vi "process mappings.vi"(4 "output dictionary":refnum<class "data dictionary.lvclass">, 6 "input dictionary":refnum<class "data dictionary.lvclass">, 8 "error in":errorcluster, 11 "modbus channels":refnum<class "Modbus Module Channel.lvclass">[](array[class])) -> (0 "error out":errorcluster, 2 "output accesses":T1[](array[typedef]), 3 "input accesses":T5[](array[typedef]))   [LabVIEW 2013, in "Modbus Slave runtime.lvclass"]
uses:
  Modbus Slave runtime.lvclass
  <vilib>/NI/Tag Bus/dictionary/data dictionary.lvclass
  bulk data access.ctl
  module channel/data bank type.ctl
  data mapping elements.ctl
  <vilib>/NI/Tag Bus/tag/Data Type.ctl
  output bulk data access.ctl
  module channel/Modbus Module Channel.lvclass
  <vilib>/NI/Tag Bus/tag/tag descriptor.lvclass
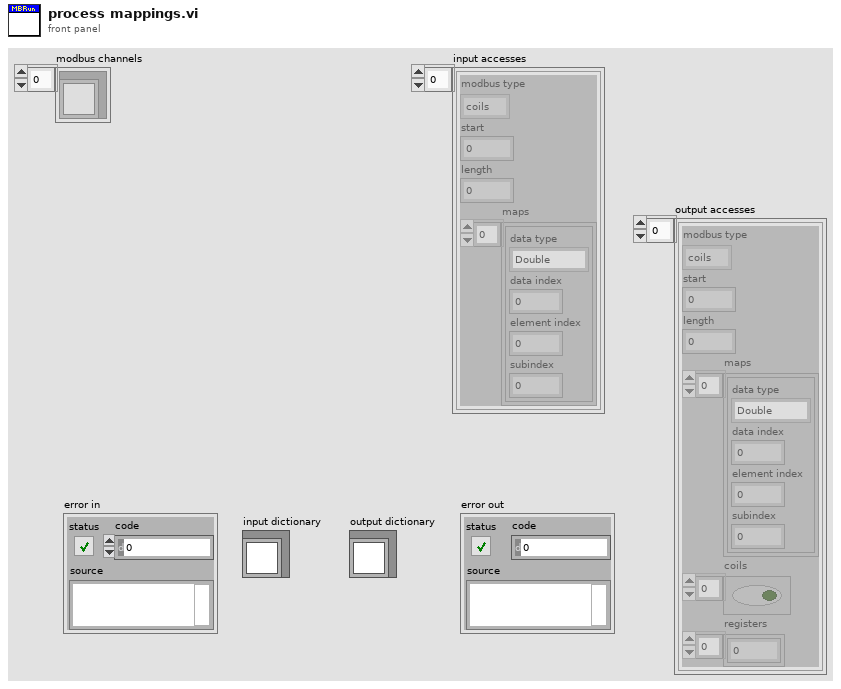
[diagram p1: front panel]
types:
  T1 = typedef "Modbus Slave runtime.lvclass/output bulk data access.ctl" = cluster{"modbus type":T2, "start":u16, "length":u16, "maps":T3[], "coils":bool[], "registers":u16[]}
  T2 = typedef "Modbus Module Channel.lvclass/data bank type.ctl" = enum16{"coils", "discrete inputs", "input registers", "holding registers"}
  T3 = typedef "Modbus Slave runtime.lvclass/data mapping elements.ctl" = cluster{"data type":T4, "data index":i32, "element index":i32, "subindex":i32}
  T4 = typedef "tag bus.lvlib/tag descriptor.lvclass/Data Type.ctl" = enum16{"Double", "Single", "I64", "I32", "I16", "I8", "U64", "U32", "U16", "U8", "Boolean", "String", "Array of Double", "Array of Single", "Array of I64", "Array of I32", "Array of I16", "Array of I8", "Array of U64", "Array of U32", "Array of U16", "Array of U8", "Array of Boolean", "Array of String"}
  T5 = typedef "Modbus Slave runtime.lvclass/bulk data access.ctl" = cluster{"modbus type":T2, "start":u16, "length":u16, "maps":T3[]}
  T6 = typedef "Modbus Slave runtime.lvclass/clump precursor.ctl" = cluster{"modbus type":T2, "channel classification":T7, "accesses":T8[]}
  T7 = typedef "TBM channel.lvclass/channel classification.ctl" = enum16{"input data", "output data", "processing parameter", "processing result"}
  T8 = typedef "Modbus Slave runtime.lvclass/clump accesses.ctl" = cluster{"starting address":u16, "last element":i32, "channel index":i32}
  T9 = typedef "Modbus Slave runtime.lvclass/clump.ctl" = cluster{"modbus type":T2, "classification":T7, "start":i32, "length":i32, "channel indices":i32[]}
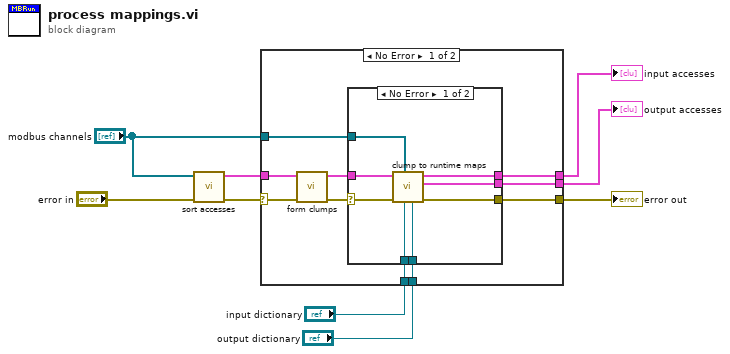
[diagram p0: block diagram]
diagram:
  n1 = call "sort accesses.vi"("error in"="error in", "modbus channels"="modbus channels") -> ("error out"=w8:errorcluster, "clump precursors"=w6:T6[])  [unwired: 8 in]
  n2 = case shown="No Error" w8 {
    selector: w8 -> [w19 w29]
    tunnel: [w16 w29] -> w7
    tunnel: w6 -> [w18 _]
    tunnel: "modbus channels" -> [w12 _]
    tunnel: "input dictionary" -> [w14 _]
    tunnel: "output dictionary" -> [w13 _]
    tunnel: [w11 _] -> w2
    tunnel: [w10 _] -> w1
    frame No Error {
      n3 = call "form clumps.vi"("error in"=w19, "clump precursors"=w18) -> ("error out"=w17:errorcluster, "clumps"=w15:T9[])  [unwired: 8 in]
      n4 = case shown="No Error" w17 {
        selector: w17 -> [w26 w28]
        tunnel: [w27 w28] -> w16
        tunnel: w15 -> [w22 _]
        tunnel: w14 -> [w20 _]
        tunnel: w13 -> [w23 _]
        tunnel: w12 -> [w21 _]
        tunnel: [w25 _] -> w11
        tunnel: [w24 _] -> w10
        frame No Error {
          n5 = call "clump to runtime maps.vi"("output dictionary"=w23, "input dictionary"=w20, "modbus channels"=w21, "error in"=w26, "clumps"=w22) -> ("error out"=w27:errorcluster, "output accesses"=w24:T1[], "input accesses"=w25:T5[])  [unwired: 4 in]
        }
        frame Error {
        }
      }
    }
    frame Error {
    }
  }
  "error out" <- w7
  "input accesses" <- w2
  "output accesses" <- w1
